vi "Control - MAP Desired.vi"(8 "Control Inputs":T1={"Engine Speed [RPM]"=0.0, "Engine Status"=enum."STALLED", "Load Control \nMode"=enum."High-Idle Governor", "dt(s)"=0.0, "Number of Cylinders"=0, "Engine Displacement [cc]"=0.0, "StoichAFR"=0.0, "Q.LHV Fuel [kJ/kg]"=0.0, "BattV PSU [V]"=0.0, "12V PSU [V]"=0.0, "5V PSU [V]"=0.0, "Pedal Position [%]"=0.0, "Oil Pressure [kPa]"=0.0, "Oil Temp [C]"=0.0, "Oil Level [%]"=0.0, "Engine Coolant Temp (ECT) [C]"=0.0, "Engine Coolant Pressure [kPa]"=0.0, "Rail Pressure [bar]"=0.0, "Fuel Pressure [kPa]"=0.0, "Fuel Temp [C]"=0.0, "Vacuum Pressure [kPa]"=0.0, "Throttle Position [%]"=0.0, "Cam1 Advance [CAD]"=0.0, "Cam2 Advance [CAD]"=0.0, "CA50 Control Output [CAD]"=[], "CA50 Control Output Valid"=[], "Intake Air Temp (IAT) [C]"=0.0, "Barometric Air Pressure [kPa]"=0.0, "Intake Air Rel. Humidity [%]"=0.0, "Mass Air Flow (MAF) [kg/hr]"=0.0, "Turbo Inlet Air Pressure [kPa]"=0.0, "Turbo Inlet Air Temp [C]"=0.0, "Turbo Outlet Air Pressure [kPa]"=0.0, "Turbo Outlet Air Temp [C]"=0.0, "CAC Outlet Pressure [kPa]"=0.0, "CAC Outlet Temp [C]"=0.0, "Intake Manifold Pressure (MAP) [kPa]"=0.0, "Intake Manifold Temp (MAT) [C]"=0.0, "Exhaust Manifold Pressure [kPa]"=0.0, "Exhaust Manifold Temp [C]"=0.0, "HighP EGR Cooler Outlet Pressure [kPa]"=0.0, "HighP EGR Cooler Outlet Temp [C]"=0.0, "HighP EGR Differential Pressure [kPa]"=0.0, "HighP EGR Valve Position [%]"=0.0, "Turbo Outlet Exhaust Pressure [kPa]"=0.0, "Turbo Outlet Exhaust Temp [C]"=0.0, "VGT Position 1 [%]"=0.0, "VGT Position 2 [%]"=0.0, "Turbo Speed 1 [RPM]"=0.0, "Turbo Speed 2 [RPM]"=0.0, "LowP EGR Differential Pressure [kPa]"=0.0, "LowP EGR Valve Position [%]"=0.0, "UEGO1Lambda"=0.0, "UEGO1_Hot"=FALSE, "UEGO2Lambda"=0.0, "UEGO2_Hot"=FALSE} {"CA50 Control Output [CAD]" format="%.2f"; "VGT Position 1 [%]" format="%.2f"; "Turbo Speed 2 [RPM]" format="%.2f"; "LowP EGR Valve Position [%]" format="%.2f"; "Turbo Inlet Air Temp [C]" format="%#_6f"; "Turbo Outlet Air Temp [C]" format="%#_6f"; "UEGO2Lambda" format="%.2f"; "Turbo Speed 1 [RPM]" format="%.2f"; "UEGO1Lambda" format="%.2f"}, 10 "Volumetric Efficiency [%]":sgl, 11 "IMEP Desired [bar]":sgl) -> (0 "Intake MAP Desired [kPa]":sgl)   [LabVIEW 2015, in "ECS-RT.lvlib"]
uses:
  ECS-RT.lvlib
  Typedefs/Control Inputs/Control Inputs.ctl
  Typedefs/EPT/Engine Status.ctl
  Typedefs/MISC/Load Control Mode.ctl
  ECS-Shared.lvlib
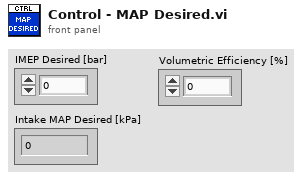
[diagram p1: front panel]
types:
  T1 = typedef "ECS-Shared.lvlib/Control Inputs.ctl" = cluster{"Engine Speed [RPM]":sgl, "Engine Status":T2, "Load Control \nMode":T3, "dt(s)":sgl, "Number of Cylinders":u8, "Engine Displacement [cc]":sgl, "StoichAFR":sgl, "Q.LHV Fuel [kJ/kg]":sgl, "BattV PSU [V]":sgl, "12V PSU [V]":sgl, "5V PSU [V]":sgl, "Pedal Position [%]":sgl, "Oil Pressure [kPa]":sgl, "Oil Temp [C]":sgl, "Oil Level [%]":sgl, "Engine Coolant Temp (ECT) [C]":sgl, "Engine Coolant Pressure [kPa]":sgl, "Rail Pressure [bar]":sgl, "Fuel Pressure [kPa]":sgl, "Fuel Temp [C]":sgl, "Vacuum Pressure [kPa]":sgl, "Throttle Position [%]":sgl, "Cam1 Advance [CAD]":sgl, "Cam2 Advance [CAD]":sgl, "CA50 Control Output [CAD]":sgl[], "CA50 Control Output Valid":bool[], "Intake Air Temp (IAT) [C]":sgl, "Barometric Air Pressure [kPa]":sgl, "Intake Air Rel. Humidity [%]":sgl, "Mass Air Flow (MAF) [kg/hr]":sgl, "Turbo Inlet Air Pressure [kPa]":sgl, "Turbo Inlet Air Temp [C]":sgl, "Turbo Outlet Air Pressure [kPa]":sgl, "Turbo Outlet Air Temp [C]":sgl, "CAC Outlet Pressure [kPa]":sgl, "CAC Outlet Temp [C]":sgl, "Intake Manifold Pressure (MAP) [kPa]":sgl, "Intake Manifold Temp (MAT) [C]":sgl, "Exhaust Manifold Pressure [kPa]":sgl, "Exhaust Manifold Temp [C]":sgl, "HighP EGR Cooler Outlet Pressure [kPa]":sgl, "HighP EGR Cooler Outlet Temp [C]":sgl, "HighP EGR Differential Pressure [kPa]":sgl, "HighP EGR Valve Position [%]":sgl, "Turbo Outlet Exhaust Pressure [kPa]":sgl, "Turbo Outlet Exhaust Temp [C]":sgl, "VGT Position 1 [%]":sgl, "VGT Position 2 [%]":sgl, "Turbo Speed 1 [RPM]":sgl, "Turbo Speed 2 [RPM]":sgl, "LowP EGR Differential Pressure [kPa]":sgl, "LowP EGR Valve Position [%]":sgl, "UEGO1Lambda":sgl, "UEGO1_Hot":bool, "UEGO2Lambda":sgl, "UEGO2_Hot":bool}
  T2 = typedef "ECS-Shared.lvlib/Engine Status.ctl" = enum16{"STALLED", "CRANKING", "RUNNING"}
  T3 = typedef "ECS-Shared.lvlib/Load Control Mode.ctl" = enum16{"No Governor", "Low-Idle Governor", "High-Idle Governor"}
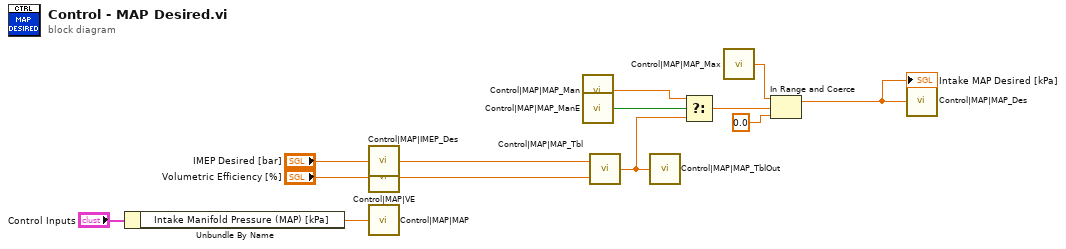
[diagram p0: block diagram]
diagram:
  n1 = Unbundle By Name("Control Inputs") -> ("Intake Manifold Pressure (MAP) [kPa]"=w7:sgl)
  n2 = call "Control|MAP|IMEP_Des"("Value"="IMEP Desired [bar]") -> ()
  n3 = call "Control|MAP|VE"("Value"="Volumetric Efficiency [%]") -> ()
  n4 = call "Control|MAP|MAP"("Value"=w7) -> ()
  n5 = call "Control|MAP|MAP_Man"() -> ("Value"=w9:sgl)
  n6 = call "Control|MAP|MAP_ManE"() -> ("Value"=w10:bool)
  n7 = call "Control|MAP|MAP_Tbl"("Y Index"="Volumetric Efficiency [%]", "X Index"="IMEP Desired [bar]") -> ("Z"=w11:sgl)
  n8 = call "Control|MAP|MAP_TblOut"("Value"=w11) -> ()
  n9 = Select(t=w9, s=w10, f=w11) -> (s? t:f=w5:sgl)
  n10 = call "Control|MAP|MAP_Max"() -> ("Value"=w3:sgl)
  n11 = In Range and Coerce(upper limit=w3, x=w5, lower limit=sgl 0.0) -> (coerced(x)=w2:sgl)  [unwired: 1 out]
  "Intake MAP Desired [kPa]" <- w2
  n12 = call "Control|MAP|MAP_Des"("Value"=w2) -> ()
